vi "Set BufferSize.vi"(8 "error in (no error)":errorcluster, 10 "Buffer Size":i32=1, 11 "CircularBuffer":refnum<class "CircularBuffer.lvclass">) -> (0 "error out":errorcluster, 3 "CircularBuffer out":refnum<class "CircularBuffer.lvclass">)   [LabVIEW 2016, in "CircularBuffer.lvclass"]
doc: "---------------------------------------------------------------\nJKI State Machine Objects™\nhttp://jki.net/state-machine-objects/\nCopyright (C) 2005-2015, JKI <info@jki.net>\nALL RIGHTS RESERVEDJKI State Machine Objects (SMO) 1.0.0.5\nJKI - JKI\nCopyright (c) 2016, JKI"
uses:
  CircularBuffer.lvclass
panel:
  # "For instructions on how to use the JKI State Machine Objects, examples and video tutorials, visit:\nhttp://jki.net/state-machine-objects/\n\nJKI State Machine Objects™\nhttp://jki.net/state-machine-objects/\nCopyright (C) 2005-2015, JKI <info@jki.net>\nALL RIGHTS RESERVED"
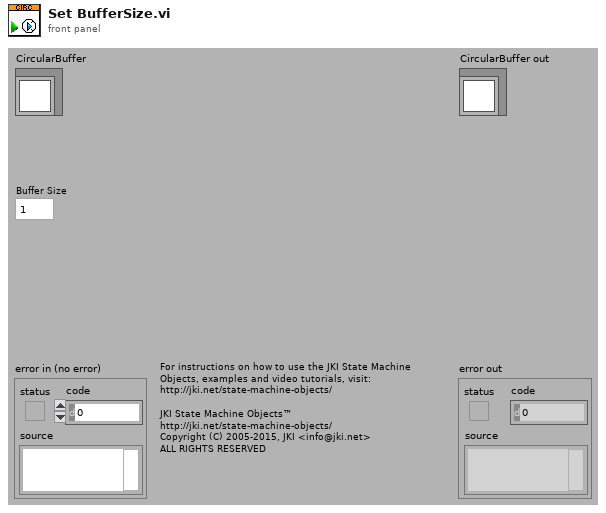
[diagram p1: front panel]
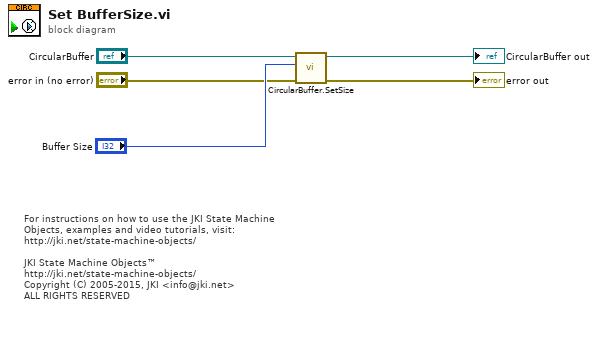
[diagram p0: block diagram]
diagram:
  # "For instructions on how to use the JKI State Machine Objects, examples and video tutorials, visit:\nhttp://jki.net/state-machine-objects/\n\nJKI State Machine Objects™\nhttp://jki.net/state-machine-objects/\nCopyright (C) 2005-2015, JKI <info@jki.net>\nALL RIGHTS RESERVED"
  n1 = call "CircularBuffer.SetSize.vi"("error in (no error)"="error in (no error)", "BufferSize"="Buffer Size", "CircularBuffer"="CircularBuffer") -> ("error out"=→"error out":errorcluster, "CircularBuffer out"=→"CircularBuffer out":refnum<class "CircularBuffer.lvclass">)  [unwired: 7 in]
